vi "test_Path.vi"() -> ()   [LabVIEW 2013]
uses:
  <vilib>/Utility/sysdir.llb/System Directory Type.ctl
  source/TypeDescriptor/TypeDescriptor_GetPString.vi
  source/TypeDescriptor/OpenDescriptor.lvlib
panel:
  out "value":string
  out "Name":string
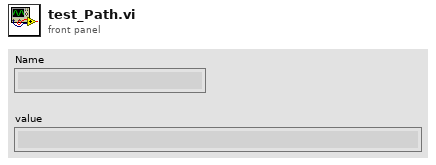
[diagram p1: front panel]
types:
  T1 = typedef "System Directory Type.ctl" = i32
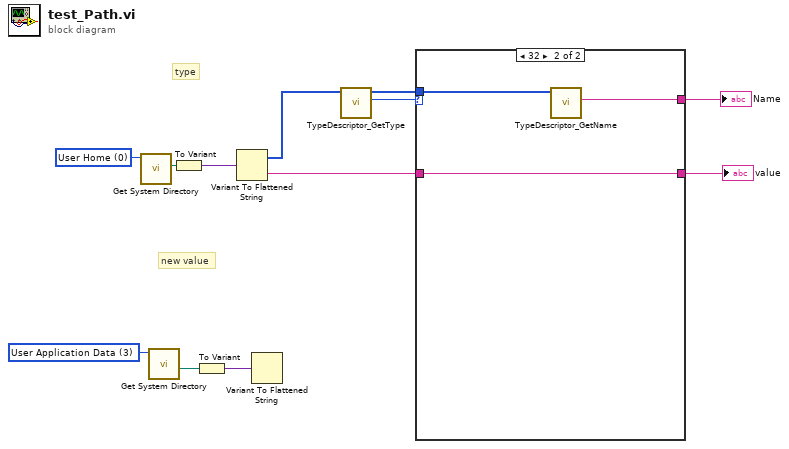
[diagram p0: block diagram]
diagram:
  w10 = T1 3 items=["User Home"=0, "User Desktop"=1, "User Documents"=2, "User Application Data"=3, "User Preferences"=4, "User Temporary"=5, "Public Documents"=6, "Public Application Data"=7, "Public Preferences"=8, "Public Cache"=13, "System Core Libraries"=9, "System Installed Libraries"=10, "Application Files"=11, "Boot Volume Root"=12] ("system directory type")
  w11 = T1 0 items=["User Home"=0, "User Desktop"=1, "User Documents"=2, "User Application Data"=3, "User Preferences"=4, "User Temporary"=5, "Public Documents"=6, "Public Application Data"=7, "Public Preferences"=8, "Public Cache"=13, "System Core Libraries"=9, "System Installed Libraries"=10, "Application Files"=11, "Boot Volume Root"=12] ("system directory type")
  # "new value"
  # "type"
  n1 = call <vilib>:"Get System Directory.vi"("system directory type"=w11) -> ("system directory"=w8:path)  [unwired: 10 in]
  n2 = call <vilib>:"Get System Directory.vi"("system directory type"=w10) -> ("system directory"=w6:path)  [unwired: 10 in]
  n3 = To Variant(anything=w8) -> (Variant=w12:variant)
  n4 = To Variant(anything=w6) -> (Variant=w7:variant)
  n5 = Variant To Flattened String(Variant=w12) -> (data string=w5:string, 1:w2:i16[])
  n6 = Variant To Flattened String(Variant=w7) -> ()  [unwired: 2 out]
  n7 = call "TypeDescriptor_GetType.vi"("type descriptor"=w2) -> ("Type"=w3:u8, "type descriptor dup"=w4:i16[])  [unwired: 9 in]
  n8 = case shown="32" w3 {
    tunnel: [_ w14] -> w9
    tunnel: w5 -> [_ w13]
    tunnel: w4 -> [_ w15]
    tunnel: [_ w13] -> w1
    frame Default {
    }
    frame 50 {
      n9 = call "TypeDescriptor_GetName.vi"("type descriptor"=w15) -> ("name"=w14:string)  [unwired: 8 in, 2 out]
    }
  }
  "Name" <- w9
  "value" <- w1
